vi "RFSG List Mode LO Signal Generation for 5668.vi"(0 "Resource Name":refnum<k15>="RFSG" caption="resource name", 1 "List Trigger Source":string(combo)="PXI_Trig1", 2 "Mode":enum16{"Normal", "Measure Flatness"}(ring), 5 "Start Frequency":dbl format="%#_6p", 7 "End Frequency":dbl format="%#_6p", 9 "Spacing":dbl=500000000.0 format="%#_13p", 11 "error in":errorcluster, 12 "output terminal":T1="PXI_Trig0") -> (4 "instrument handle out":refnum<k15>, 15 "error out":errorcluster)   [LabVIEW 2017]
doc: "Demonstrates how to create a Configuration List for sweeping frequency and/or power."
uses:
  <instrlib>/niRFSG/niRFSG.llb/niRFSG Exported Signal Destinations.ctl
  <instrlib>/niRFSG/niRFSG.llb/niRFSG Configuration List Properties.ctl
  <instrlib>/niRFSG/niRFSG.llb/niRFSG Signal Names.ctl
  <instrlib>/niRFSG/niRFSG.llb/niRFSG Ref Clock Sources.ctl
panel:
  # "Overview: Demonstrates how to create a Configuration List for sweeping frequency and/or power.\nRequirements: NI-RFSG\nInstructions:\n1. Change the Resource Name to your device.\n2. Run the VI.\n3. Click Stop to stop the VI."
  # "In order to configure new settings, you must stop the example using \nthe Stop button and then run the VI with the new settings."
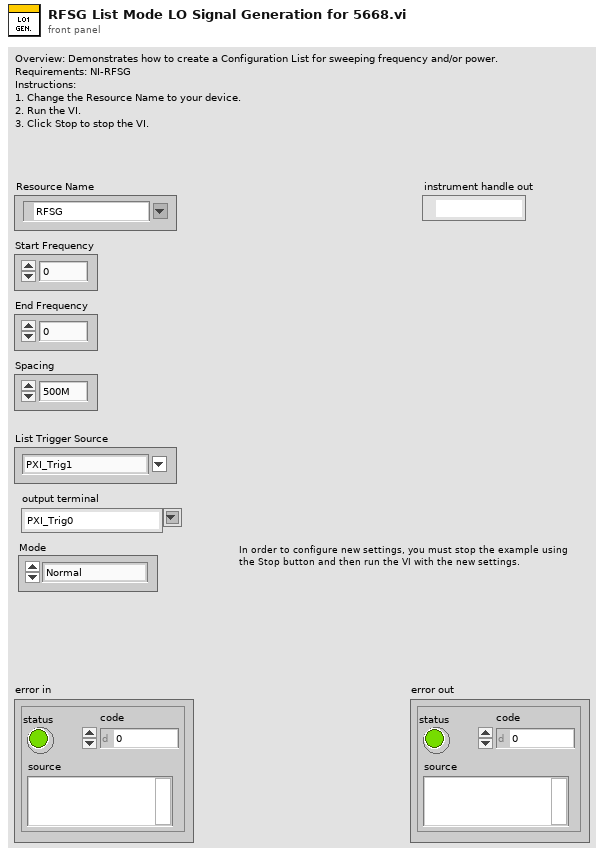
[diagram p1: front panel]
types:
  T1 = typedef "niRFSG Exported Signal Destinations.ctl" = string
  T2 = typedef "niRFSG Ref Clock Sources.ctl" = string
  T3 = typedef "niRFSG Signal Names.ctl" = i32
  T4 = typedef "niRFSG Configuration List Properties.ctl" = u32
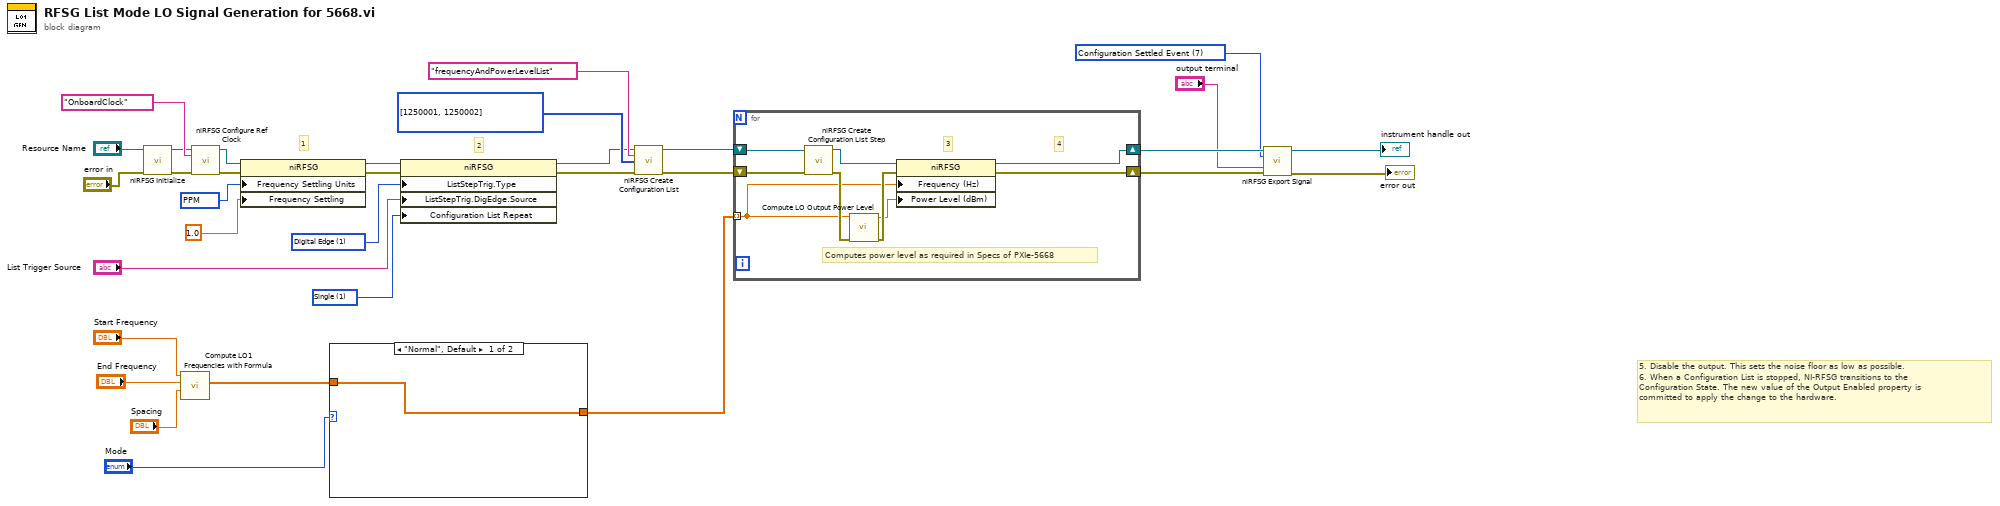
[diagram p0: block diagram]
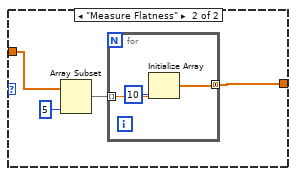
[diagram p2: hidden frame]
diagram:
  w10 = 1 items=["Continuous", "Single"] ("Configuration List:Configuration List Repeat")
  w11 = T3 7 items=["Start Trigger", "Script Trigger", "Marker Event", "Ref Clock", "Started Event", "Done Event", "Configuration List Step Trigger", "Configuration Settled Event"] ("signal")
  w23 = T4[] [1250001, 1250002] items=["ALC Control"=1150195, "Amp Path"=1150185, "Amplitude Settling (dB)"=1150137, "Attenuator Setting (dB)"=1150173, "Automatic Power Search"=1150196, "Frequency (Hz)"=1250001, "Frequency Settling"=1150083, "IQ Out Port Carrier Frequency"=1150145, "IQ Out Port Common Mode Offset"=1150148, "IQ Out Port Level"=1150147, "IQ Out Port Offset"=1150149, "Output Enabled"=1250004, "Phase Offset (Degrees)"=1150024, "Power Level (dBm)"=1250002, "Pulse Modulation Enabled"=1250051, "Timer Event Interval (s)"=1150100, "Upconverter Center Frequency (Hz)"=1154098] ("configuration list properties")
  w30 = 1 items=["None", "Digital Edge", "Software"] ("Triggers:Configuration List Step:Type")
  w32 = 12002 items=["Seconds After Lock"=12000, "Seconds After I/O"=12001, "PPM"=12002] ("RF:Frequency Settling Units")
  # "2"
  # "5. Disable the output. This sets the noise floor as low as possible.\n6. When a Configuration List is stopped, NI-RFSG transitions to the Configuration State. The new value of the Output Enabled property is committed to apply the change to the hardware."
  # "1"
  n1 = call <instrlib>:"niRFSG Initialize.vi"("resource name"="Resource Name", "error in"="error in") -> ("instrument handle"=w18:refnum<k15>, "error out"=w17:errorcluster)  [unwired: 2 in, 10 out]
  n2 = call "Compute LO1 Frequencies with Formula.vi"("Spacing"="Spacing", "Stop Frequency"="End Frequency", "Start Frequency"="Start Frequency") -> ("LO1 Frequencies"=w3:dbl[])  [unwired: 6 in, 2 out]
  n3 = call <instrlib>:"niRFSG Configure Ref Clock.vi"("instrument handle"=w18, "ref clock source"=T2 "OnboardClock" ("Reference Clock Source"), "error in"=w17) -> ("instrument handle out"=w20:refnum<k15>, "error out"=w21:errorcluster)  [unwired: 1 in, 10 out]
  n4 = property class="niRFSG"(reference=w20, error in=w21, "Frequency Settling Units"=w32, "Frequency Settling"=1.0 ("Frequency Settling (ppm)")) -> (reference out=w27:refnum<k15>, error out=w28:errorcluster)
  n5 = case shown="\"Normal\", Default" "Mode" {
    tunnel: w3 -> [w33 w37]
    tunnel: [w33 w34] -> w2
    frame "Normal", Default {
    }
    frame "Measure Flatness" {
      n6 = Array Subset(array=w37, length=5) -> (w35:dbl[])  [unwired: 1 in]
      n7 = for {
        tunnel: w35 -> [w39] mode=indexing
        tunnel: [w38] -> w34 mode=concatenating
        n8 = Initialize Array(w39, 10 ("dimension size")) -> (w38:dbl[])
      }
    }
  }
  n9 = property class="niRFSG"(reference=w27, error in=w28, "ListStepTrig.Type"=w30, "ListStepTrig.DigEdge.Source"="List Trigger Source", "Configuration List Repeat"=w10) -> (reference out=w19:refnum<k15>, error out=w24:errorcluster)
  n10 = call <instrlib>:"niRFSG Create Configuration List.vi"("instrument handle"=w19, "list name"="frequencyAndPowerLevelList", "configuration list properties"=w23, "error in"=w24) -> ("instrument handle out"=w16:refnum<k15>, "error out"=w29:errorcluster)  [unwired: 1 in, 9 out]
  n11 = for {
    shift-right: [w47] -> w14
    shift-left: w16 -> [w43]
    shift-right: [w48] -> w13
    shift-left: w29 -> [w42]
    tunnel: w2 -> [w41] mode=indexing
    # "Computes power level as required in Specs of PXIe-5668"
    # "4"
    # "3"
    n12 = call <instrlib>:"niRFSG Create Configuration List Step.vi"("instrument handle"=w43, "error in"=w42) -> ("instrument handle out"=w49:refnum<k15>, "error out"=w46:errorcluster)  [unwired: 1 in, 11 out]
    n13 = call "Compute LO Output Power Level.vi"("error in"=w46, "LO1 Frequency (Hz)"=w41) -> ("error out"=w45:errorcluster, "Power Level"=w44:dbl)  [unwired: 8 in]
    n14 = property class="niRFSG"(reference=w49, error in=w45, "Frequency (Hz)"=w41, "Power Level (dBm)"=w44) -> (reference out=w47:refnum<k15>, error out=w48:errorcluster)
  }
  n15 = call <instrlib>:"niRFSG Export Signal.vi"("instrument handle"=w14, "signal"=w11, "output terminal"="output terminal", "error in"=w13) -> ("instrument handle out"=→"instrument handle out":refnum<k15>, "error out"=→"error out":errorcluster)  [unwired: 10 in]
